vi "QGSettings.vi"(1 "Set/Get":bool, 2 "QG Settings (input)":T1={"channels (trigger)"="2", "Trigger Amplitude (V)"=0.0} {"Trigger Amplitude (V)" format="%.2f"}) -> (0 "QG Settings (output)":T1={"channels (trigger)"="2", "Trigger Amplitude (V)"=0.0} {"Trigger Amplitude (V)" format="%.2f"})   [LabVIEW 2009]
uses:
  QGSettings.ctt
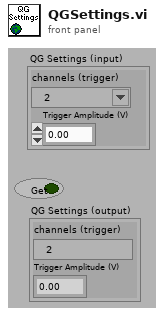
[diagram p1: front panel]
types:
  T1 = typedef "QGSettings.ctt" = cluster{"channels (trigger)":tag, "Trigger Amplitude (V)":dbl}
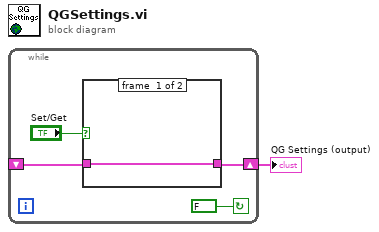
[diagram p0: block diagram]
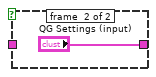
[diagram p2: hidden frame]
diagram:
  n1 = while {
    shift-right: [w3] -> w1
    shift-left: _ -> [w4]
    stop <- FALSE continue-if-true
    n2 = case shown="True" "Set/Get" {
      tunnel: [w6 "QG Settings (input)"] -> w3
      tunnel: w4 -> [w6 _]
      frame #0 {
      }
      frame #1 {
      }
    }
  }
  "QG Settings (output)" <- w1
